vi "DAQmx Create Channel (TEDS-AI-Temperature-Thermistor-Vex).vi"(0 "task in":refnum<k21>, 1 "maximum value":dbl=100.0 format="%0.2f", 2 "minimum value":dbl format="%0.2f", 3 "resistance configuration":i32(ring)=4 items=["2-Wire"=2, "3-Wire"=3, "4-Wire"=4], 5 "physical channels":tag, 7 "name to assign":string, 9 "units":i32(ring)=10143 items=["Deg C"=10143, "Deg F"=10144, "Kelvins"=10325, "Deg R"=10145, "From Custom Scale"=10065], 10 "voltage excitation value":dbl=2.5 format="%0.5f", 11 "error in":errorcluster, 13 "voltage excitation source":i32(ring)=10167 items=["Internal"=10200, "External"=10167, "None"=10230], 14 "r1":dbl=5000.0 format="%0.2f") -> (4 "task out":refnum<k21>, 15 "error out":errorcluster)   [LabVIEW 2018]
doc: "Creates channel(s) that use a thermistor to measure temperature. Use this instance when the thermistor requires voltage excitation. You must configure the physical channel(s) with TEDS information to use this VI."
uses:
  nilvaiu.dll
panel:
  # "input limits"
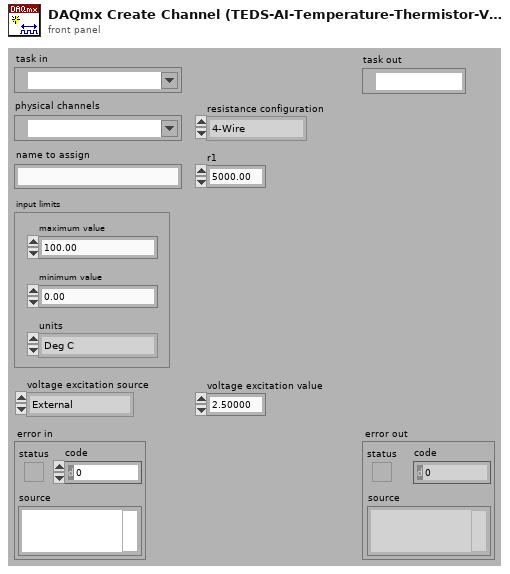
[diagram p1: front panel]
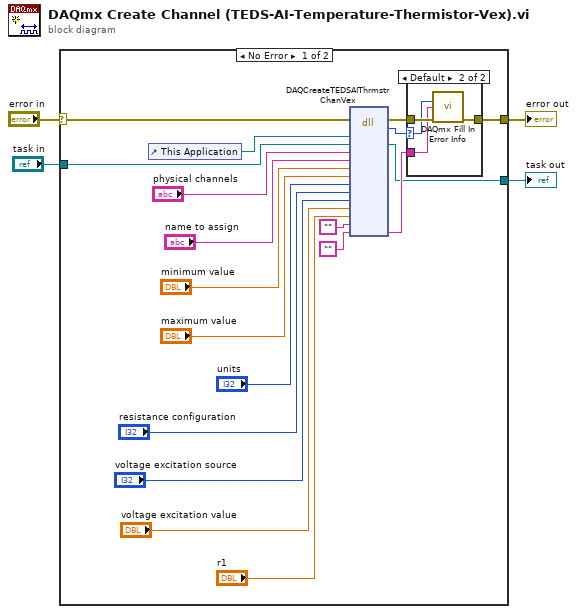
[diagram p0: block diagram]
diagram:
  n1 = case shown="No Error" "error in" {
    selector: "error in" -> [w8 w29]
    tunnel: "task in" -> [w10 w30]
    tunnel: [w9 w30] -> w3
    tunnel: [w7 w29] -> w1
    frame No Error {
      n2 = control-ref of="This Application"() -> (w21:refnum<vi>)
      n3 = dll-call lib="nilvaiu.*" fn="DAQCreateTEDSAIThrmstrChanVex"(error in=w8, "lvAppRef"=w21, "refObjPtr"=w10, "physicalChannelName"="physical channels", "channelNameIn"="name to assign", "minVal"="minimum value", "maxVal"="maximum value", "units"="units", "resistanceConfig"="resistance configuration", "voltageExcitSource"="voltage excitation source", "voltageExcitVal"="voltage excitation value", "r1"="r1", "channelNamesOut"="", "extendedErrorInfo"="") -> (error out=w23:errorcluster, "return type"=w22:i32, "refObjPtr"=w9:refnum<k21>, "extendedErrorInfo"=w11:string)  [unwired: 13 in, 1 out]
      n4 = case shown="Default" w22 {
        selector: w22 -> [_ w26]
        tunnel: w23 -> [w24 w28]
        tunnel: [w24 w27] -> w7
        tunnel: w11 -> [_ w25]
        frame 0 {
        }
        frame Default {
          n5 = call "DAQmx Fill In Error Info.vi"("status code"=w26, "extended error info"=w25, "error in"=w28) -> ("error out"=w27:errorcluster)  [unwired: 1 in, 11 out]
        }
      }
    }
    frame Error {
    }
  }
  "task out" <- w3
  "error out" <- w1
